vi "Read Home Status.vi"(8 "error in (no error)":errorcluster, 11 "Axis in":refnum<class "Axis.lvclass">) -> (0 "error out":errorcluster, 2 "Home?":bool, 3 "Axis out":refnum<class "Axis.lvclass">)   [LabVIEW 2018, in "Axis.lvlib" / "Axis.lvclass"]
uses:
  Axis.lvclass
  Axis.lvclass/Axis.ctl
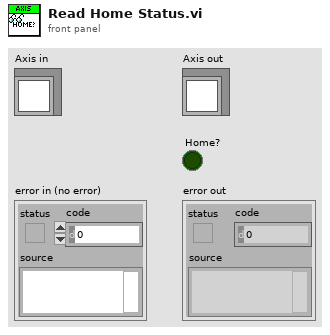
[diagram p1: front panel]
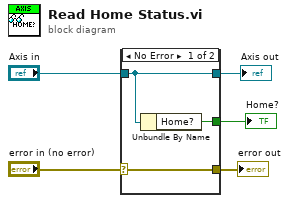
[diagram p0: block diagram]
diagram:
  n1 = case shown="No Error" "error in (no error)" {
    selector: "error in (no error)" -> [w8 w9]
    tunnel: [w8 w9] -> w4
    tunnel: [w7 w10] -> w2
    tunnel: "Axis in" -> [w7 w10]
    tunnel: [w6 _] -> w1
    frame No Error {
      n2 = Unbundle By Name(w7) -> ("Home?"=w6:bool)
    }
    frame Error {
    }
  }
  "error out" <- w4
  "Axis out" <- w2
  "Home?" <- w1
